vi "梦幻城堡C6~20界面.vi"() -> ()   [LabVIEW 2016, in "环境动力监测库.lvlib" / "UPS库.lvlib"]
uses:
  <vilib>/Utility/config.llb/NI_LVConfig.lvlib
  <vilib>/ptbypt/NI_PtbyPt.lvlib
panel:
  out "关闭中":bool
  out "关机倒计时":i32
  out "UPS状态":T1
  out "K":dbl
  out "CCC":dbl
  out "通信指示":bool
  in  "关机":bool
  in  "重开串口":bool
  out "Temperature":dbl
  out "Battery voltage":dbl
  out "I/P frequency HZ":dbl
  out "O/P load %":dbl
  out "O/P voltage":dbl
  out "I/P voltage":dbl
  # "UPS-梦幻城堡C6~20"
  # "输入电压V"
  # "输出电压V"
  # "输出电流A"
  # "输入频率HZ"
  # "电池电压V"
  # "UPS温度℃"
  # "电池容量百分比"
  # "系统模式"
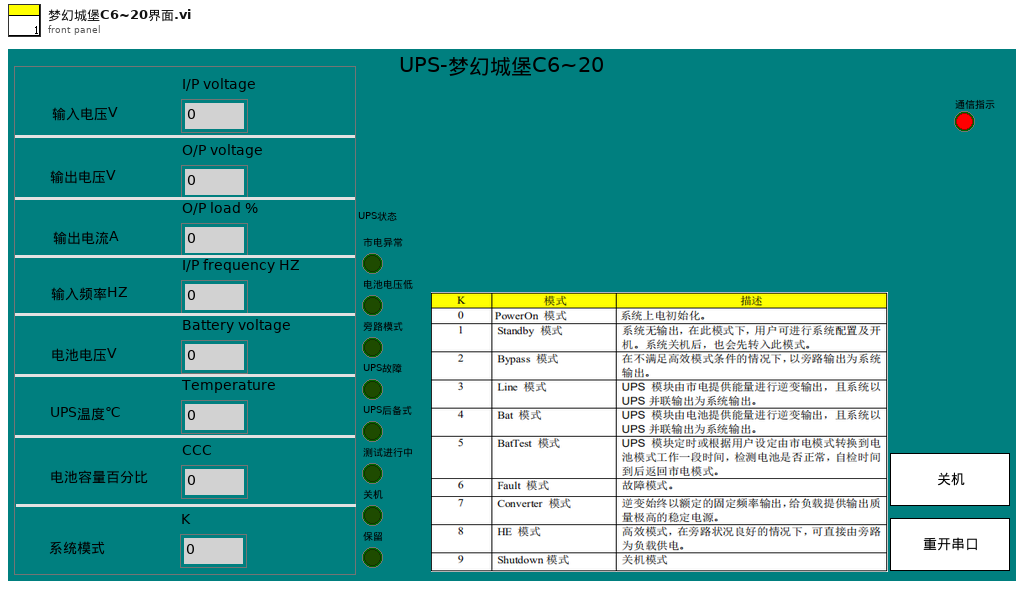
[diagram p1: front panel]
types:
  T1 = cluster{"市电异常":bool, "电池电压低":bool, "旁路模式":bool, "UPS故障":bool, "UPS后备式":bool, "测试进行中":bool, "关机":bool, "保留":bool}
  T2 = cluster{"枚举":enum16{"open", "read", "write", "close"}, "写入缓冲区":string}
  T3 = cluster{"时间标识":timestamp, "设备":string, "日志信息":string}
  T4 = typedef "NI_LVConfig.lvlib/Config Data RefNum.ctl" = refnum<k1>
  T5 = cluster{"输出功率R":dbl, "输出功率S":dbl, "输出功率T":dbl, "输出视在功率R":dbl, "输出视在功率S":dbl, "输出视在功率T":dbl, "总功率":dbl, "总视在功率":dbl, "输出电流R":dbl, "输出电流S":dbl, "输出电流T":dbl, "输出负载百分比":dbl, "U":string}
  T6 = cluster{"输入电压R":dbl, "输入电压S":dbl, "输入电压T":dbl, "输入频率":dbl, "输出电压R":dbl, "输出电压S":dbl, "输出电压T":dbl, "输出频率":dbl, "输出电流R":dbl, "输出电流S":dbl, "输出电流T":dbl, "Positive电池电压":dbl, "Negative电池电压":dbl, "温度":dbl, "电池剩余备用时间":dbl, "电池容量百分比":dbl, "系统模式":dbl, "电池测试状态":dbl, "故障代码":string, "告警":string}
  T7 = cluster{"[0]":bool, "[1]":bool, "[2]":bool, "[3]":bool, "[4]":bool, "[5]":bool, "[6]":bool, "[7]":bool}
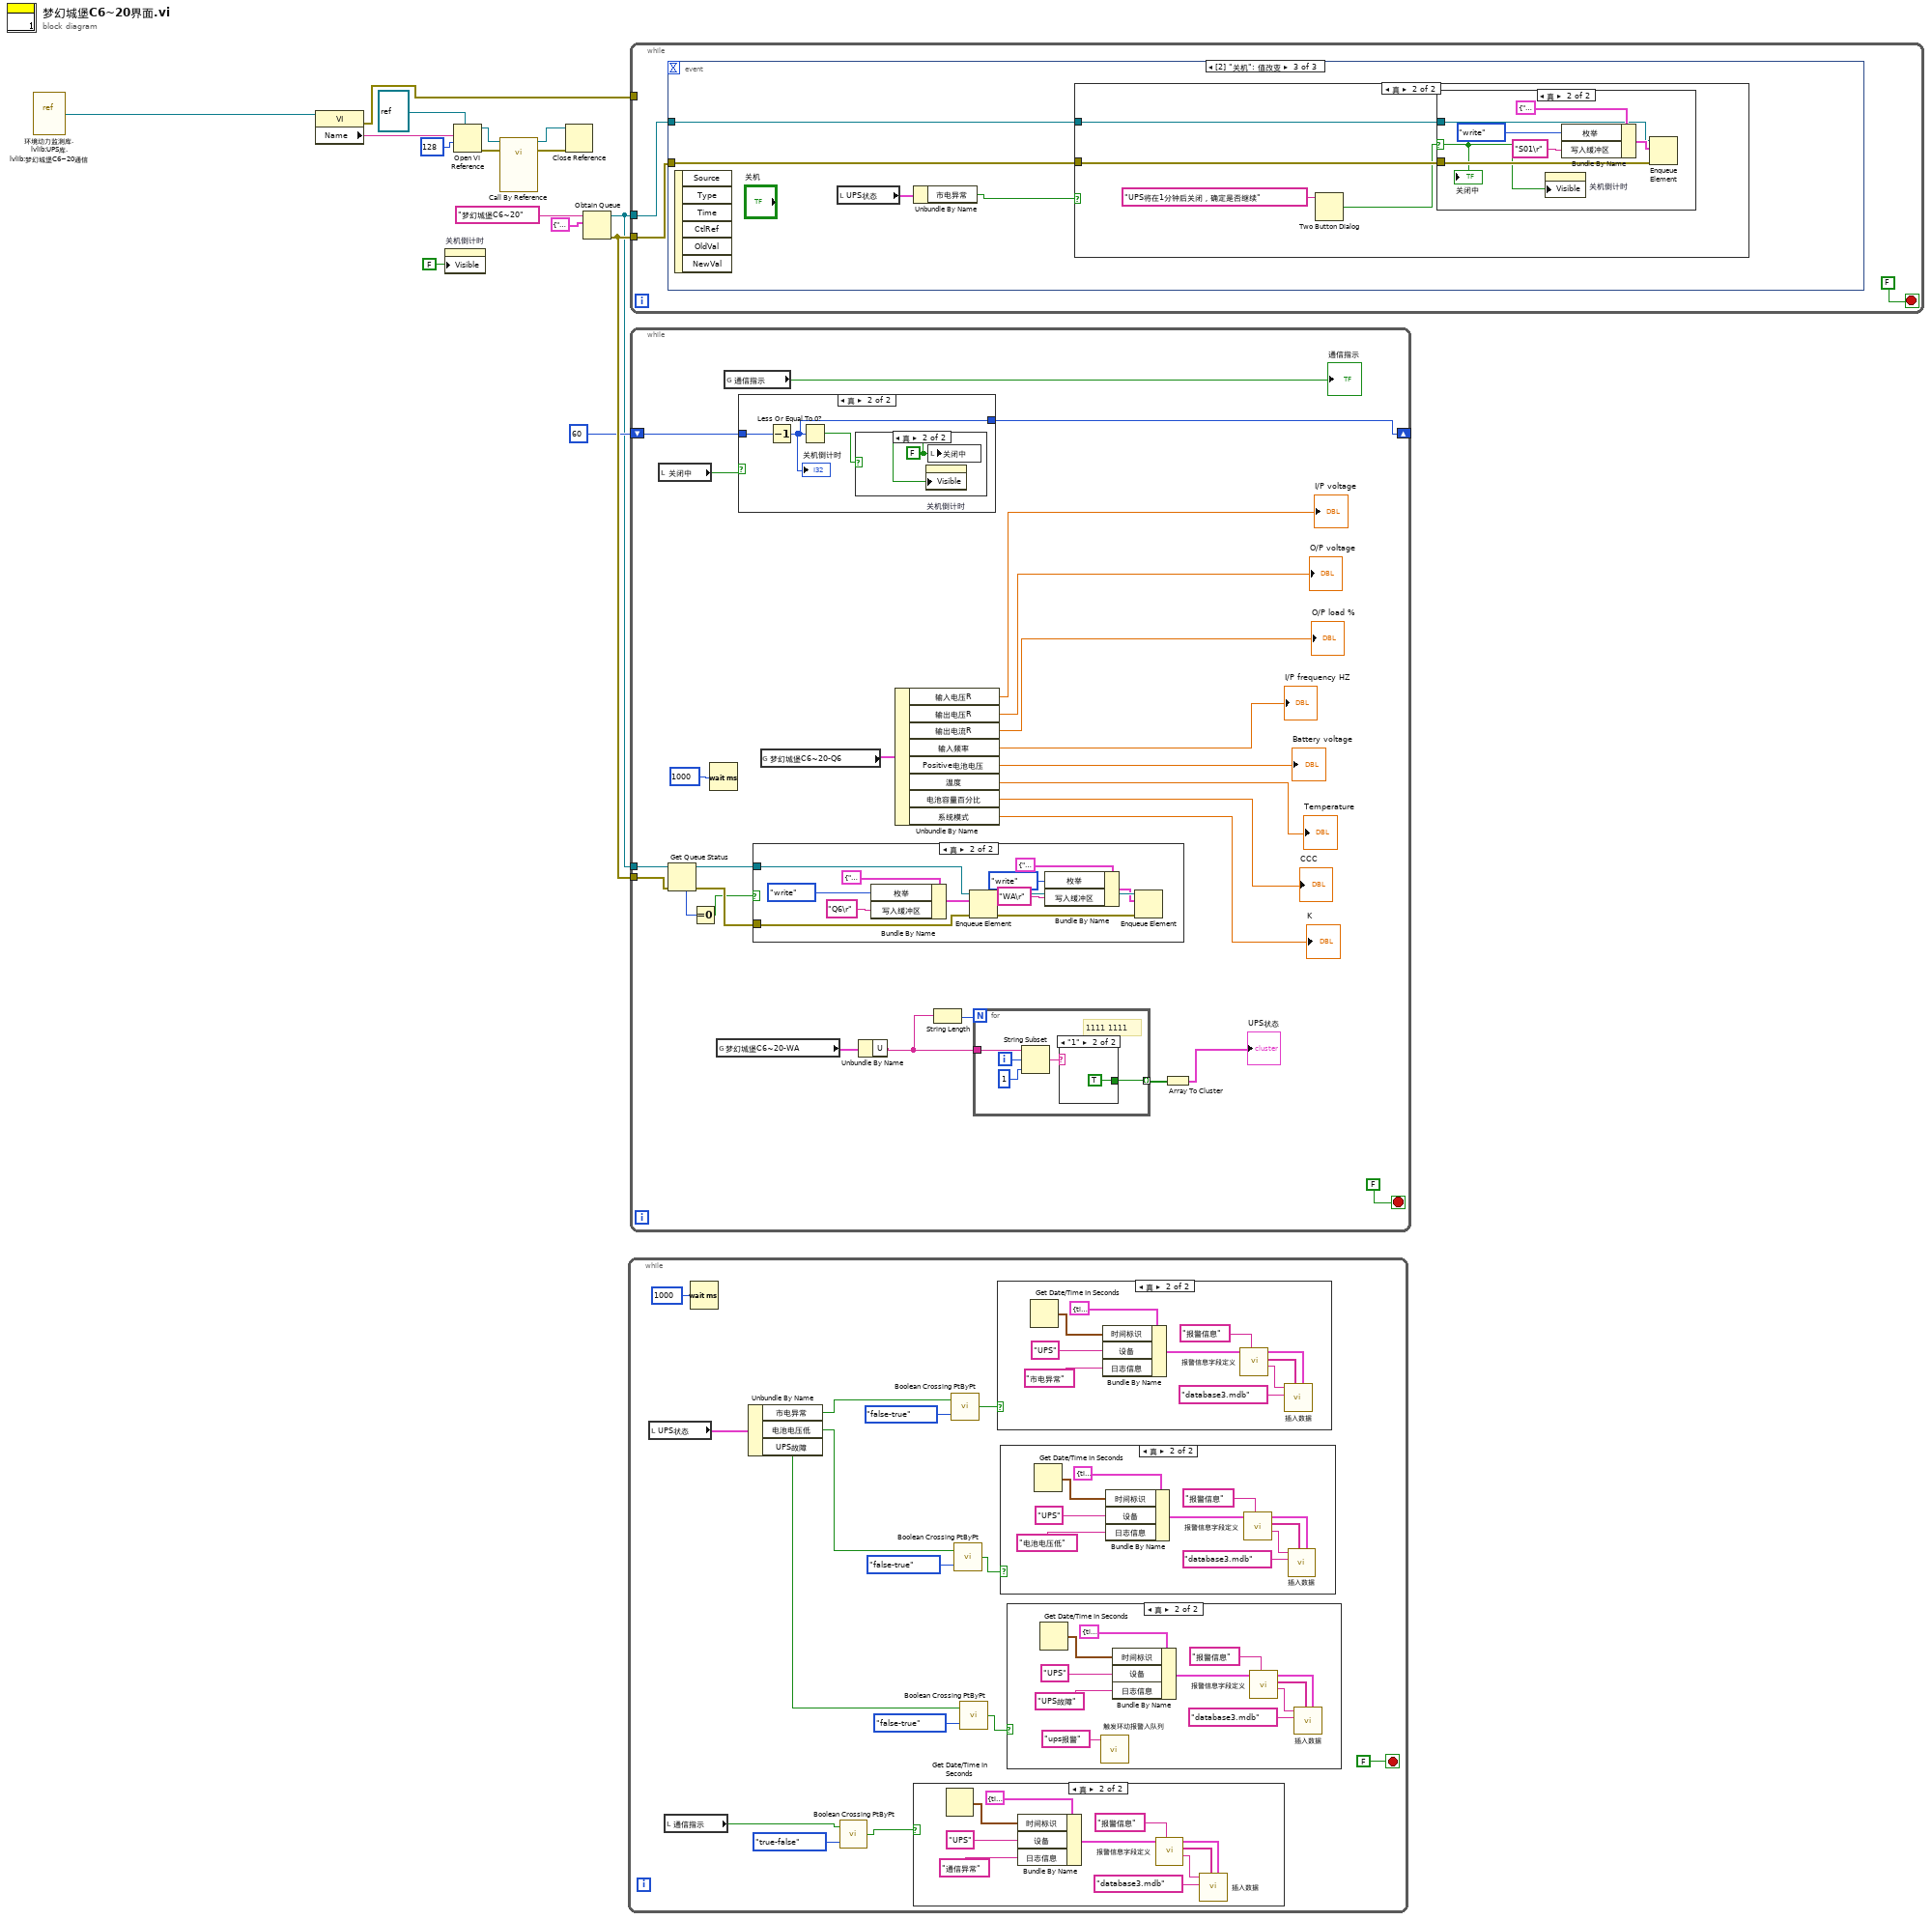
[diagram p0: block diagram]
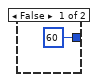
[diagram p6: hidden frame]
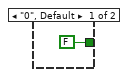
[diagram p8: hidden frame]
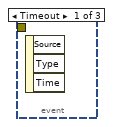
[diagram p10: hidden frame]
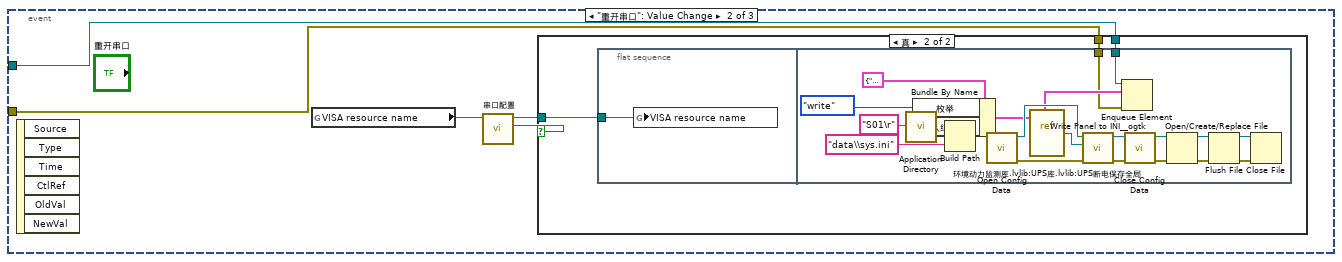
[diagram p11: hidden frame]
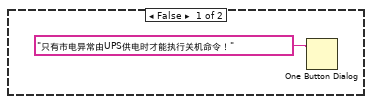
[diagram p13: hidden frame]
diagram:
  n1 = vi-ref "环境动力监测库.lvlib:UPS库.lvlib:梦幻城堡C6~20通信.vi"() -> (w8:refnum<vi>)
  n2 = property class="VI"(reference=w8) -> (error out=w2:errorcluster, "Name"=w9:string)  [unwired: 1 in, 1 out]
  n3 = property on="关机倒计时" class="DigNum (严格)"("Visible"=FALSE ("可见")) -> ()  [unwired: 2 in, 2 out]
  n4 = Open VI Reference(type specifier VI Refnum (for type only)=refnum<vi> refnum, vi path=w9, options=128 ("选项")) -> (vi reference=w11:refnum<vi>, error out=w13:errorcluster)  [unwired: 3 in]
  n5 = call-by-ref "?"(reference=w11, error in=w13) -> (reference out=w15:refnum<vi>, error out=w14:errorcluster)  [unwired: 12 in]
  n6 = Close Reference(reference=w15, error in (no error)=w14) -> ()  [unwired: 1 out]
  n7 = Obtain Queue(name (unnamed)="梦幻城堡C6~20" ("名称（未命名）"), element data type=T2 {"枚举"=enum."open", "写入缓冲区"=""}) -> (queue out=w3:refnum<queue>, error out=w5:errorcluster)  [unwired: 3 in, 1 out]
  n8 = while {
    stop <- FALSE stop-if-true
    n9 = local read "UPS状态"() -> (w20:T1)
    n10 = local read "通信指示"() -> (w17:bool)
    n11 = Wait (ms)(milliseconds to wait=u32 1000 ("等待时间（毫秒）")) -> ()  [unwired: 1 out]
    n12 = Unbundle By Name(w20) -> ("市电异常"=w27:bool, "电池电压低"=w22:bool, "UPS故障"=w21:bool)
    n13 = call <vilib>:"Boolean Crossing PtByPt.vi"("direction"=enum16{"either", "false-true", "true-false"}."true-false", "input"=w17) -> ("crossing"=w16:bool)  [unwired: 1 in]
    n14 = case shown="真" w16 {
      frame False {
      }
      frame True {
        n15 = Get Date/Time In Seconds() -> (seconds since 1Jan1904=w39:timestamp)
        n16 = Bundle By Name(cluster=T3 {"时间标识"=timestamp(0 s since 1904-01-01), "设备"="", "日志信息"=""} ("data in"), "时间标识"=w39, "设备"="UPS", "日志信息"="通信异常") -> (w38:T3)
        n17 = call "报警信息字段定义.vi"("table输入"="报警信息", "data in"=w38) -> ("table输出"=w34:string, "columns"=w33:string[], "data out"=w32:T3)  [unwired: 7 in]
        n18 = call "插入数据.vi"("data"=w32, "columns"=w33, "database"="database3.mdb", "table"=w34) -> ()  [unwired: 7 in, 1 out]
      }
    }
    n19 = call <vilib>:"Boolean Crossing PtByPt.vi"("direction"=enum16{"either", "false-true", "true-false"}."false-true", "input"=w27) -> ("crossing"=w28:bool)  [unwired: 1 in]
    n20 = call <vilib>:"Boolean Crossing PtByPt.vi"("direction"=enum16{"either", "false-true", "true-false"}."false-true", "input"=w22) -> ("crossing"=w25:bool)  [unwired: 1 in]
    n21 = call <vilib>:"Boolean Crossing PtByPt.vi"("direction"=enum16{"either", "false-true", "true-false"}."false-true", "input"=w21) -> ("crossing"=w24:bool)  [unwired: 1 in]
    n22 = case shown="真" w28 {
      frame False {
      }
      frame True {
        n23 = Get Date/Time In Seconds() -> (seconds since 1Jan1904=w70:timestamp)
        n24 = Bundle By Name(cluster=T3 {"时间标识"=timestamp(0 s since 1904-01-01), "设备"="", "日志信息"=""} ("data in"), "时间标识"=w70, "设备"="UPS", "日志信息"="市电异常") -> (w69:T3)
        n25 = call "报警信息字段定义.vi"("table输入"="报警信息", "data in"=w69) -> ("table输出"=w65:string, "columns"=w64:string[], "data out"=w63:T3)  [unwired: 7 in]
        n26 = call "插入数据.vi"("data"=w63, "columns"=w64, "database"="database3.mdb", "table"=w65) -> ()  [unwired: 7 in, 1 out]
      }
    }
    n27 = case shown="真" w25 {
      frame False {
      }
      frame True {
        n28 = Get Date/Time In Seconds() -> (seconds since 1Jan1904=w60:timestamp)
        n29 = Bundle By Name(cluster=T3 {"时间标识"=timestamp(0 s since 1904-01-01), "设备"="", "日志信息"=""} ("data in"), "时间标识"=w60, "设备"="UPS", "日志信息"="电池电压低") -> (w59:T3)
        n30 = call "报警信息字段定义.vi"("table输入"="报警信息", "data in"=w59) -> ("table输出"=w55:string, "columns"=w54:string[], "data out"=w53:T3)  [unwired: 7 in]
        n31 = call "插入数据.vi"("data"=w53, "columns"=w54, "database"="database3.mdb", "table"=w55) -> ()  [unwired: 7 in, 1 out]
      }
    }
    n32 = case shown="真" w24 {
      frame False {
      }
      frame True {
        n33 = Get Date/Time In Seconds() -> (seconds since 1Jan1904=w50:timestamp)
        n34 = call "触发环动报警入队列.vi"("报警内容"="ups报警") -> ()  [unwired: 11 in]
        n35 = Bundle By Name(cluster=T3 {"时间标识"=timestamp(0 s since 1904-01-01), "设备"="", "日志信息"=""} ("data in"), "时间标识"=w50, "设备"="UPS", "日志信息"="UPS故障") -> (w49:T3)
        n36 = call "报警信息字段定义.vi"("table输入"="报警信息", "data in"=w49) -> ("table输出"=w45:string, "columns"=w44:string[], "data out"=w43:T3)  [unwired: 7 in]
        n37 = call "插入数据.vi"("data"=w43, "columns"=w44, "database"="database3.mdb", "table"=w45) -> ()  [unwired: 7 in, 1 out]
      }
    }
  }
  n38 = while {
    tunnel: w5 -> [w73]
    tunnel: w3 -> [w72]
    tunnel: w2 -> [_]
    stop <- FALSE stop-if-true
    n39 = event shown="[2] \"关机\": 值改变" {
      selector: _ -> [_ _ _]
      dyn-events: _ -> [_ _ _]
      timeout: _ -> [_ _ _]
      tunnel: w73 -> [_ w75 w106]
      tunnel: w72 -> [_ w76 w107]
      event Timeout {
        n40 = event-data() -> ()  [unwired: 1 in, 3 out]
      }
      event "重开串口": Value Change {
        n41 = event-data() -> ()  [unwired: 1 in, 6 out]
        n42 = global read "UPS断电保存全局.vi" "VISA resource name"() -> (w79:refnum<visa-resource-name>)
        n43 = call "串口配置.vi"("请选择串口:"=w79) -> ("确认 2"=w78:bool, "请选择串口: 2"=w77:refnum<visa-resource-name>)  [unwired: 9 in]
        n44 = case shown="真" w78 {
          tunnel: w77 -> [_ w82]
          tunnel: w76 -> [_ w81]
          tunnel: w75 -> [_ w80]
          frame False {
          }
          frame True {
            n45 = flat-sequence {
              tunnel: w82 -> [w83]
              tunnel: w81 -> [w85]
              tunnel: w80 -> [w84]
              frame #0 {
                n46 = global write "UPS断电保存全局.vi" "VISA resource name"(w83) -> ()
              }
              frame #1 {
                n47 = call <vilib>:"Application Directory.vi"() -> ("Application Directory"=w91:path)
                n48 = Bundle By Name(cluster=T2 {"枚举"=enum."open", "写入缓冲区"=""}, "枚举"=enum16{"open", "read", "write", "close"}."write" ("元素"), "写入缓冲区"="S01\r") -> (w89:T2)
                n49 = Build Path(base path=w91, name or relative path="data\\sys.ini" ("名称或相对路径")) -> (appended path=w92:path)
                n50 = call <vilib>:"Open Config Data.vi"("configuration file path"=w92) -> ("error out"=w96:errorcluster, "refnum"=w93:T4)  [unwired: 8 in, 1 out]
                n51 = vi-ref "环境动力监测库.lvlib:UPS库.lvlib:UPS断电保存全局.vi"() -> (w94:refnum<vi>)
                n52 = call <userlib>:"Write Panel to INI__ogtk.vi"("error in (no error)"=w96, "VI ref"=w94, "refnum"=w93) -> ("error out"=w97:errorcluster, "refnum out"=w95:T4)  [unwired: 7 in]
                n53 = Enqueue Element(queue=w85, element=w89, error in (no error)=w84) -> ()  [unwired: 1 in, 3 out]
                n54 = call <vilib>:"Close Config Data.vi"("error in (no error)"=w97, "refnum"=w95) -> ("error out"=w102:errorcluster, "file path"=w103:path)  [unwired: 8 in]
                n55 = Open/Create/Replace File(file path (use dialog)=w103, error in=w102) -> (refnum out=w99:refnum<file>, error out=w98:errorcluster)  [unwired: 4 in, 1 out]
                n56 = Flush File(refnum=w99, error in=w98) -> (refnum out=w100:refnum<file>, error out=w101:errorcluster)
                n57 = Close File(refnum=w100, error in=w101) -> ()  [unwired: 2 out]
              }
            }
          }
        }
      }
      event "关机": Value Change {
        n58 = event-data() -> ()  [unwired: 1 in, 6 out]
        n59 = local read "UPS状态"() -> (w105:T1)
        n60 = Unbundle By Name(w105) -> ("市电异常"=w104:bool)
        n61 = case shown="真" w104 {
          tunnel: w107 -> [_ w112]
          tunnel: w106 -> [_ w111]
          frame False {
            n62 = One Button Dialog(message="只有市电异常由UPS供电时才能执行关机命令！" ("消息")) -> ()  [unwired: 1 in, 1 out]
          }
          frame True {
            n63 = Two Button Dialog(message="UPS将在1分钟后关闭，确定是否继续" ("消息")) -> (T button?=w109:bool)  [unwired: 2 in]
            n64 = case shown="真" w109 {
              selector: w109 -> [_ w113]
              tunnel: w112 -> [_ w116]
              tunnel: w111 -> [_ w115]
              frame False {
              }
              frame True {
                n65 = property on="关机倒计时" class="DigNum (严格)"("Visible"=w113) -> ()  [unwired: 2 in, 2 out]
                n66 = Bundle By Name(cluster=T2 {"枚举"=enum."open", "写入缓冲区"=""}, "枚举"=enum16{"open", "read", "write", "close"}."write", "写入缓冲区"="S01\r") -> (w117:T2)
                n67 = Enqueue Element(queue=w116, element=w117, error in (no error)=w115) -> ()  [unwired: 1 in, 3 out]
                "关闭中" <- w113
              }
            }
          }
        }
      }
    }
  }
  n68 = while {
    tunnel: w3 -> [w133]
    tunnel: w5 -> [w132]
    shift-right: [w120] -> _
    shift-left: 60 -> [w121]
    stop <- FALSE stop-if-true
    n69 = local read "关闭中"() -> (w122:bool)
    n70 = Get Queue Status(queue=w133, error in (no error)=w132) -> (queue out=w131:refnum<queue>, error out=w130:errorcluster, # elements in queue=w129:i32)  [unwired: 1 in, 5 out]
    n71 = Equal To 0?(x=w129) -> (x = 0?=w128:bool)
    n72 = Wait (ms)(milliseconds to wait=u32 1000 ("等待时间（毫秒）")) -> ()  [unwired: 1 out]
    n73 = global read "UPS内部交互全局.vi" "梦幻城堡C6~20-WA"() -> (w127:T5)
    n74 = global read "UPS内部交互全局.vi" "通信指示"() -> (→"通信指示":bool)
    n75 = case shown="真" w122 {
      tunnel: w121 -> [_ w149]
      tunnel: [60 w148] -> w120
      frame False {
      }
      frame True {
        n76 = Decrement(x=w149) -> (x-1=w148:i32)
        "关机倒计时" <- w148
        n77 = Less Or Equal To 0?(x=w148) -> (x <= 0?=w147:bool)
        n78 = case shown="真" w147 {
          frame False {
          }
          frame True {
            w150 = FALSE ("关闭中")
            n79 = property on="关机倒计时" class="DigNum (严格)"("Visible"=w150) -> ()  [unwired: 2 in, 2 out]
            n80 = local write "关闭中"(w150) -> ()
          }
        }
      }
    }
    n81 = case shown="真" w128 {
      tunnel: w131 -> [_ w165]
      tunnel: w130 -> [_ w164]
      frame False {
      }
      frame True {
        n82 = Bundle By Name(cluster=T2 {"枚举"=enum."open", "写入缓冲区"=""}, "枚举"=enum16{"open", "read", "write", "close"}."write", "写入缓冲区"="Q6\r") -> (w168:T2)
        n83 = Enqueue Element(queue=w165, element=w168, error in (no error)=w164) -> (queue out=w163:refnum<queue>, error out=w162:errorcluster)  [unwired: 1 in, 1 out]
        n84 = Bundle By Name(cluster=T2 {"枚举"=enum."open", "写入缓冲区"=""}, "枚举"=enum16{"open", "read", "write", "close"}."write", "写入缓冲区"="WA\r") -> (w158:T2)
        n85 = Enqueue Element(queue=w163, element=w158, error in (no error)=w162) -> ()  [unwired: 1 in, 3 out]
      }
    }
    n86 = global read "UPS内部交互全局.vi" "梦幻城堡C6~20-Q6"() -> (w143:T6)
    n87 = Unbundle By Name(w127) -> ("U"=w124:string)
    n88 = Unbundle By Name(w143) -> ("输入电压R"=→"I/P voltage":dbl, "输出电压R"=→"O/P voltage":dbl, "输出电流R"=→"O/P load %":dbl, "输入频率"=→"I/P frequency HZ":dbl, "Positive电池电压"=→"Battery voltage":dbl, "温度"=→"Temperature":dbl, "电池容量百分比"=→"CCC":dbl, "系统模式"=→"K":dbl)
    n89 = String Length(string=w124) -> (length=w126:i32)
    n90 = for {
      N: w126 -> [_]
      tunnel: w124 -> [w155]
      tunnel: [w151] -> w125 mode=indexing
      i -> [w153]
      # "1111 1111"
      n91 = String Subset(string=w155, offset (0)=w153, length (rest)=1 ("长度（剩余）")) -> (substring=w152:string)
      n92 = case shown="\"1\"" w152 {
        tunnel: [FALSE TRUE] -> w151
        frame "0", Default {
        }
        frame "1" {
        }
      }
    }
    n93 = Array To Cluster(array=w125) -> (cluster=→"UPS状态":T7)
  }
